vi "Interpret Licor RawData.vi"(11 "Licor Rawdata":string[](array[string])) -> (0 "remain":string[](array[string]), 1 "log":string[][](array[string]), 2 "calibration data out":dbl[][](array[numeric]), 3 "source data out":dbl[][](array[numeric]))   [LabVIEW 2010]
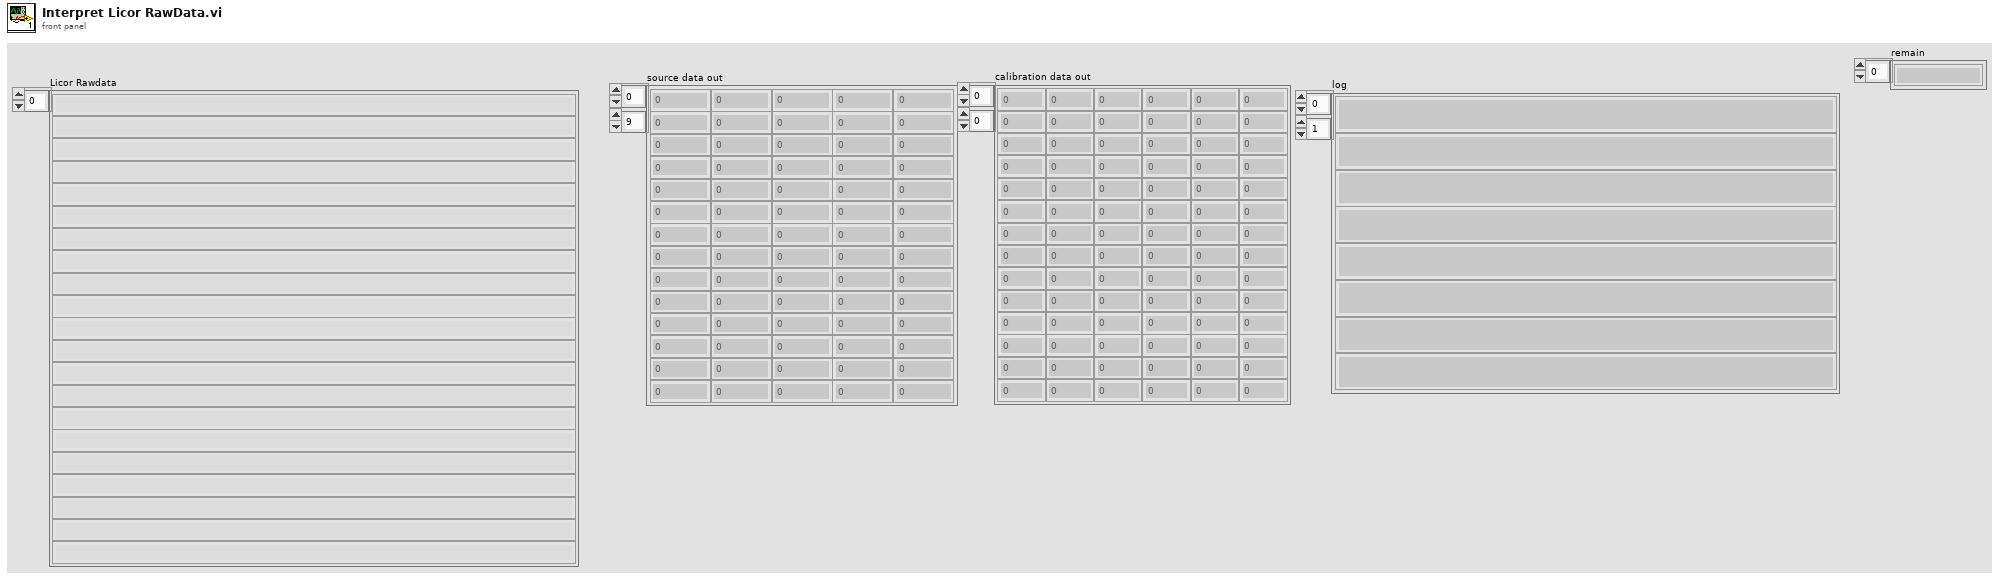
[diagram p1: front panel]
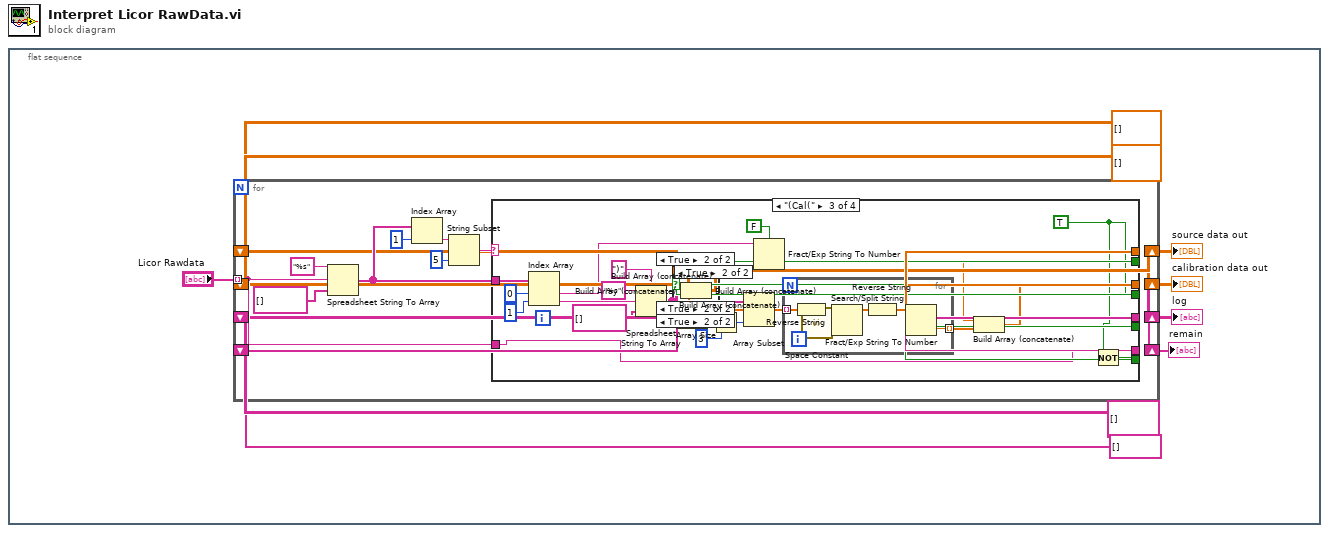
[diagram p0: block diagram]
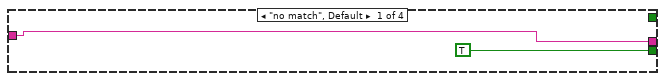
[diagram p6: hidden frame]
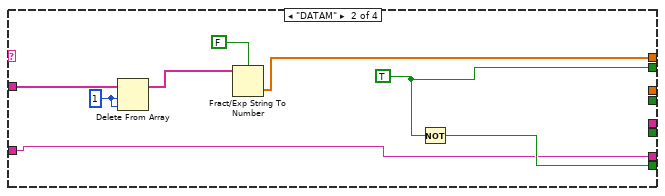
[diagram p7: hidden frame]
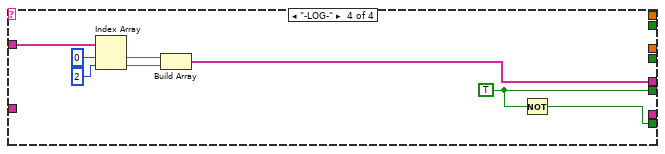
[diagram p8: hidden frame]
diagram:
  n1 = flat-sequence {
    frame #0 {
      n2 = for {
        tunnel: "Licor Rawdata" -> [w18] mode=indexing
        shift-right: [w16] -> w9
        shift-left: dbl[][] [] ("Array") -> [w17]
        shift-right: [w14] -> w8
        shift-left: dbl[][] [] ("Array") -> [w15]
        shift-right: [w12] -> w7
        shift-left: string[][] [] ("Array") -> [w13]
        shift-right: [w10] -> w5
        shift-left: string[] [] ("Array") -> [w11]
        n3 = Spreadsheet String To Array(format string="%s", spreadsheet string=w18, array type (2D Dbl)=string[] []) -> (array=w19:string[])  [unwired: 1 in]
        n4 = Index Array(array=w19, index=1 ("Index")) -> (element=w26:string)
        n5 = String Subset(string=w26, length (rest)=5 ("Länge (Rest)")) -> (substring=w32:string)  [unwired: 1 in]
        n6 = case shown="\"(Cal(\"" w32 {
          tunnel: [_ _ w66 _] -> w29
          tunnel: [_ w52 _ _] -> w31
          tunnel: [_ w56 _ _] -> w30
          tunnel: [_ _ w64 _] -> w28
          tunnel: w19 -> [_ w59 w70 w91]
          tunnel: [_ _ _ w88] -> w25
          tunnel: [w50 w55 w63 _] -> w24
          tunnel: [_ _ _ w87] -> w23
          tunnel: [TRUE w57 w65 w86] -> w22
          tunnel: w18 -> [w50 w55 w63 _]
          frame "no match", Default {
          }
          frame "DATAM" {
            w56 = TRUE
            w58 = 1 ("Länge")
            n7 = Delete From Array(array=w59, length=w58, index=w58) -> (array with subset deleted=w54:string[])  [unwired: 1 out]
            n8 = Fract/Exp String To Number(use system decimal point (T)=FALSE ("Systemdezimalzeichen verwenden (T)"), string=w54) -> (number=w52:dbl[])  [unwired: 2 in, 1 out]
            n9 = Not(x=w56) -> (.not. x?=w57:bool)
          }
          frame "(Cal(" {
            w64 = TRUE
            n10 = Index Array(array=w70, index #1=0 ("Index"), index #2=1 ("Index")) -> (element #1=w62:string, element #2=w67:string)
            n11 = Spreadsheet String To Array(delimiter (Tab)=")" ("Trennzeichen (Tabulator)"), format string="%s" ("Format-String"), spreadsheet string=w67, array type (2D Dbl)=string[] []) -> (array=w75:string[])
            n12 = Array Size(array=w75) -> (size(s)=w76:i32)
            n13 = Subtract(x=w76, y=3) -> (x-y=w78:i32)
            n14 = Array Subset(array=w75, length=w78) -> (w79:string[])  [unwired: 1 in]
            n15 = Fract/Exp String To Number(use system decimal point (T)=FALSE ("Systemdezimalzeichen verwenden (T)"), string=w62) -> (number=w61:dbl)  [unwired: 2 in, 1 out]
            n16 = for {
              tunnel: w79 -> [w83] mode=indexing
              tunnel: [w84] -> w71 mode=indexing
              n17 = Reverse String(1:w83) -> (0:w82:string)
              n18 = call <vilib>:"Space Constant.vi"() -> ("String"=w85:string)
              n19 = Search/Split String(string=w82, search string/char (-)=w85) -> (substring before match=w81:string)  [unwired: 1 in, 2 out]
              n20 = Reverse String(1:w81) -> (0:w80:string)
              n21 = Fract/Exp String To Number(string=w80) -> (number=w84:dbl)  [unwired: 3 in, 1 out]
            }
            n22 = Build Array (concatenate)(w61, w71) -> (w66:dbl[])
            n23 = Not(x=w64) -> (.not. x?=w65:bool)
          }
          frame "-LOG-" {
            w87 = TRUE
            n24 = Index Array(array=w91, index #1=0 ("Index"), index #2=2 ("Index")) -> (element #1=w90:string, element #2=w89:string)
            n25 = Build Array(w90, w89) -> (w88:string[])
            n26 = Not(x=w87) -> (.not. x?=w86:bool)
          }
        }
        n27 = case shown="True" w22 {
          tunnel: w11 -> [w34 w36]
          tunnel: w24 -> [_ w35]
          tunnel: [w34 w37] -> w10
          frame False {
          }
          frame True {
            n28 = Build Array (concatenate)(w36, w35) -> (w37:string[])
          }
        }
        n29 = case shown="True" w23 {
          tunnel: w13 -> [w38 w40]
          tunnel: w25 -> [_ w39]
          tunnel: [w38 w41] -> w12
          frame False {
          }
          frame True {
            n30 = Build Array (concatenate)(w40, w39) -> (w41:string[][])
          }
        }
        n31 = case shown="True" w28 {
          tunnel: w15 -> [w42 w44]
          tunnel: w29 -> [_ w43]
          tunnel: [w42 w45] -> w14
          frame False {
          }
          frame True {
            n32 = Build Array (concatenate)(w44, w43) -> (w45:dbl[][])
          }
        }
        n33 = case shown="True" w30 {
          tunnel: w17 -> [w46 w48]
          tunnel: w31 -> [_ w47]
          tunnel: [w46 w49] -> w16
          frame False {
          }
          frame True {
            n34 = Build Array (concatenate)(w48, w47) -> (w49:dbl[][])
          }
        }
      }
      "calibration data out" <- w8
      "source data out" <- w9
      "log" <- w7
      "remain" <- w5
    }
  }
